vi "RPMToRadps.vi"(1 "rpm":dbl) -> (0 "rad/s":dbl)   [LabVIEW 2018]
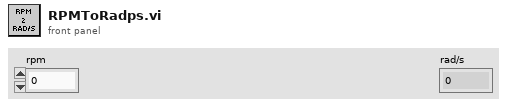
[diagram p1: front panel]
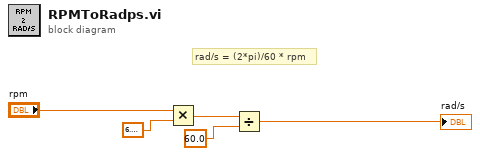
[diagram p0: block diagram]
diagram:
  # "rad/s = (2*pi)/60 * rpm"
  n1 = Multiply(x="rpm", y=6.283185307179586) -> (x*y=w4:dbl)
  n2 = Divide(x=w4, y=60.0) -> (x/y=→"rad/s":dbl)
